vi "Quaternion_Get_LVQuat.vi"(11 "Quaternion":T2={"R"=1.0, "V"=[0.0, 0.0, 0.0]}) -> (3 "LV Quaternion":T1)   [LabVIEW 2019, in "Trajectory_Library.lvlib"]
doc: "Convert a Quaternion to a LabVIEW formatted quaternion data structure (array).\n\nParameters:\n - Quaternion - The quaternion data cluster.\n\nReturns:\n - LV Quaternion - The LabVIEW quaternion"
uses:
  Trajectory_Library.lvlib
  TypeDef/QUATERNION.ctl
  <vilib>/robotics/Kinematics/Quaternion.ctl
  <vilib>/robotics/Kinematics/NI_Kinematics.lvlib
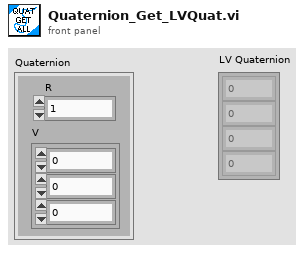
[diagram p1: front panel]
types:
  T1 = typedef "NI_Kinematics.lvlib/Quaternion.ctl" = dbl[]
  T2 = typedef "Trajectory_Library.lvlib/QUATERNION.ctl" = cluster{"R":dbl, "V":dbl[]}
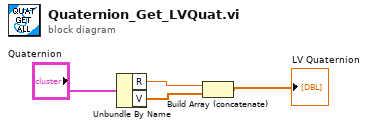
[diagram p0: block diagram]
diagram:
  n1 = Unbundle By Name("Quaternion") -> ("R"=w3:dbl, "V"=w2:dbl[])
  n2 = Build Array (concatenate)(w3, w2) -> (→"LV Quaternion":dbl[])
